vi "Read Digital Data.vi"(6 "Keyword Name":string, 7 "Section Name":string, 8 "error in (no error)":errorcluster, 10 "DigNum Refnum":refnum<vi>, 11 "file refnum":T1) -> (0 "error out":errorcluster)   [LabVIEW 2013]
uses:
  <vilib>/Utility/config.llb/Config Data RefNum.ctl
  <vilib>/Utility/config.llb/Read Key (String).vi
  <vilib>/Utility/config.llb/NI_LVConfig.lvlib
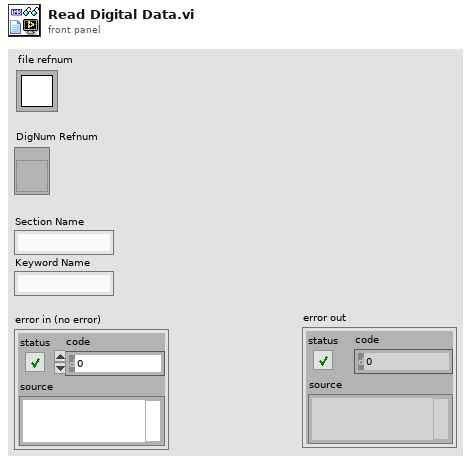
[diagram p1: front panel]
types:
  T1 = typedef "NI_LVConfig.lvlib/Config Data RefNum.ctl" = refnum<k1>
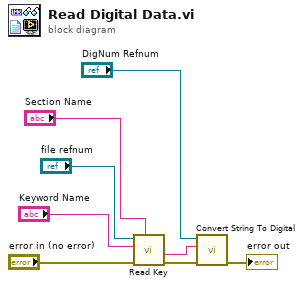
[diagram p0: block diagram]
diagram:
  n1 = call-poly <vilib>:"Read Key.vi"("section"="Section Name", "error in (no error)"="error in (no error)", "key"="Keyword Name", "refnum"="file refnum") -> ("error out"=w6:errorcluster, "value"=w1:string)  [unwired: 4 in, 2 out]
  n2 = call "Convert String To Digital.vi"("error in (no error)"=w6, "Value"=w1, "DigNum Refnum"="DigNum Refnum") -> ("error out"=→"error out":errorcluster)  [unwired: 8 in]
